vi "Preview_Build.vi"(8 "error in (no error)":errorcluster, 11 "Build in":refnum<class "AB_Targetfile.lvclass">) -> (0 "error out":errorcluster, 1 "GeneratedFiles":path[](array[path]), 3 "Build out":refnum<class "AB_Targetfile.lvclass">, 4 "GeneratedFileGUIDs":string[](array[string]), 5 "OutputDirectory":path)   [LabVIEW 2020, in "AB_Targetfile.lvclass"]
uses:
  <vilib>/AppBuilder/AB_Classes/TargetFile/AB_Targetfile.lvclass
  e:/builds/penguin/labview/branches/2020/dev/dist/vi.lib/AppBuilder/AB_Classes/Build/AB_Build.lvclass
  <vilib>/AppBuilder/AB_Classes/Build/AB_Build.lvclass
  <vilib>/AppBuilder/AB_Classes/Destination/AB_Destination.lvclass
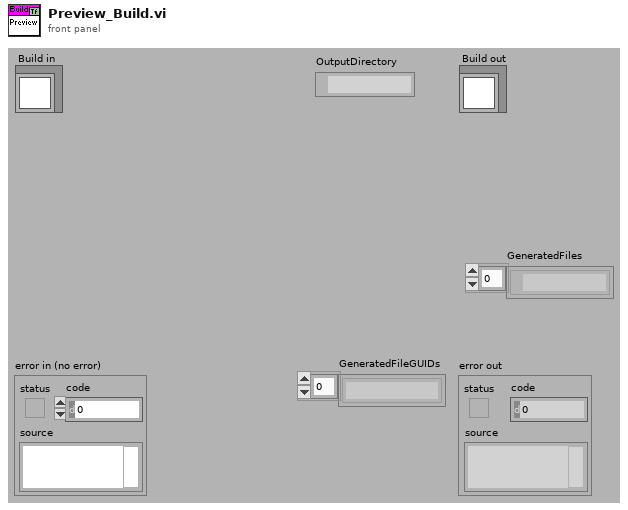
[diagram p1: front panel]
types:
  T1 = enum32{"invalid OS target", "Mac OS", "Windows 3.1", "Windows 95/NT", "Solaris 1", "Solaris 2", "HP-UX", "PowerMAX", "Linux", "Irix", "Rhapsody", "BeOS", "AIX", "OSF1", "VxWorks", "PharLap", "Carbon", "RTX", "Windows x64", "Linux x64", "Mac OS X x64"}
  T2 = typedef "AB_Build.ctl" = cluster{"buildSpecName":string, "buildSpecDescription":string, "destinations":refnum<class "AB_Destination.lvclass">[], "exclusionOption":T3, "defaultLanguage":string, "supportedLanguages":string[], "excludedDirectories":path[], "buildContext":refnum<vi>, "buildObject":T4, "preview":bool, "programatic":bool, "progressBarEvents":T5, "userLog_Path":path, "preActionID":string, "preAction_Path":path, "postActionID":string, "postAction_Path":path, "eng_checkForBrokenVIs?":bool, "eng_verboseLinkerErrors?":bool, "localDest_Path":path, "targetDest_Path":path, "removeVIObject":u16, "cache":refnum<class "PreviewCache.lvclass">, "use cache":bool, "previewCache_ID":string, "buildCache_ID":string, "eng_TempLocalDest_Path":path, "eng_collectDependencies?":bool, "versionInfo":cluster{"buildVersion":cluster{"major":u16, "minor":u16, "patch":u16, "build":u16}, "autoIncrement":bool}, "eng_enableVIChecksums":bool}
  T3 = typedef "AB_Exclusion_Option.ctl" = cluster{"typedefs":bool, "polymorphicVIs":bool, "unusedLibraryItems":bool, "modifyLibraryFile":bool, "edit-timeDependencies":bool, "inlineVIs":bool, "dependent PPLs":bool, "dependent DLLs":bool}
  T4 = typedef "ItemRef.ctl" = u64
  T5 = typedef "provcom_ProgressBar_Events.ctl" = cluster{"newJob":refnum<user-event>, "newItem":refnum<user-event>, "errorMsg":T6, "cancel":refnum<user-event>}
  T6 = typedef "mxLvBuildError.ctl" = refnum<user-event>
  T7 = typedef "AB_Destination.ctl" = cluster{"destName":string, "path":path, "libraryName":string, "preserveHierarchy":bool, "eng_inBuild":bool, "eng_libraryReference":refnum<vi>, "eng_restictAddToNewLibrary":bool}
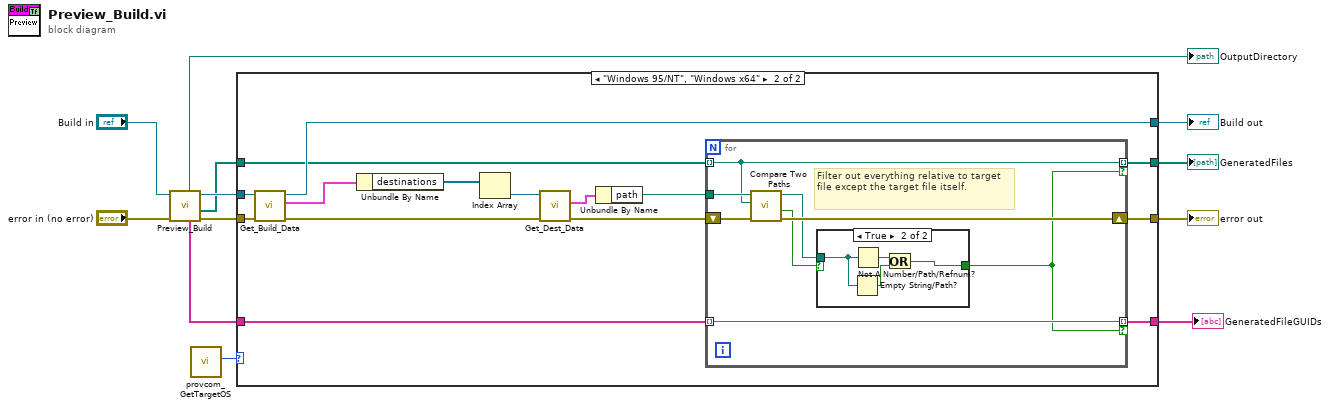
[diagram p0: block diagram]
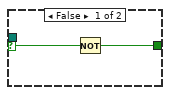
[diagram p3: hidden frame]
diagram:
  n1 = call-parent "Preview_Build.vi"("error in (no error)"="error in (no error)", "Build in"="Build in") -> ("error out"=w7:errorcluster, "GeneratedFiles"=w5:path[], "Build out"=w9:refnum<class "AB_Targetfile.lvclass">, "GeneratedFileGUIDs"=w2:string[], "OutputDirectory"=→"OutputDirectory":path)  [unwired: 5 in]
  n2 = call <resource>:"provcom_GetTargetOS.vi"() -> ("App.TargetOS"=w1:T1)  [unwired: 11 out]
  n3 = case shown="\"Windows 95/NT\", \"Windows x64\"" w1 {
    tunnel: w9 -> [w16 w31]
    tunnel: [w16 w30] -> w8
    tunnel: w7 -> [w14 w29]
    tunnel: [w14 w21] -> w6
    tunnel: w5 -> [w15 w20]
    tunnel: [w15 w19] -> w4
    tunnel: [w13 w18] -> w3
    tunnel: w2 -> [w13 w17]
    frame Default {
    }
    frame "Windows 95/NT", "Windows x64" {
      n4 = call <vilib>:"Get_Build_Data.vi"("error in (no error)"=w29, "Class in"=w31) -> ("error out"=w25:errorcluster, "data"=w28:T2, "Class out"=w30:refnum<class "AB_Targetfile.lvclass">)  [unwired: 7 in]
      n5 = Unbundle By Name(w28) -> ("destinations"=w27:refnum<class "AB_Destination.lvclass">[])
      n6 = Index Array(array=w27) -> (element=w26:refnum<class "AB_Destination.lvclass">)  [unwired: 1 in]
      n7 = call <vilib>:"Get_Dest_Data.vi"("error in (no error)"=w25, "Class in"=w26) -> ("error out"=w22:errorcluster, "destName"=w24:T7)  [unwired: 7 in, 1 out]
      n8 = Unbundle By Name(w24) -> ("path"=w23:path)
      n9 = for {
        tunnel: w23 -> [w39]
        shift-right: [w37] -> w21
        shift-left: w22 -> [w38]
        tunnel: w20 -> [w36] mode=indexing
        tunnel: [w36] -> w19 mode=indexing if=w32
        tunnel: w17 -> [w33] mode=indexing
        tunnel: [w33] -> w18 mode=indexing if=w32
        # "Filter out everything relative to target file except the target file itself."
        n10 = call <vilib>:"Compare Two Paths.vi"("error in (no error)"=w38, "Path 2"=w36, "Path 1"=w39) -> ("error out"=w37:errorcluster, "Path 2 Relative to Path 1?"=w34:bool, "Relative Path from 1 to 2"=w35:path)  [unwired: 5 in, 1 out]
        n11 = case shown="True" w34 {
          selector: w34 -> [w41 _]
          tunnel: w35 -> [_ w45]
          tunnel: [w40 w42] -> w32
          frame False {
            n12 = Not(x=w41) -> (.not. x?=w40:bool)
          }
          frame True {
            n13 = Empty String/Path?(string/path=w45) -> (empty?=w43:bool)
            n14 = Not A Number/Path/Refnum?(number/path/refnum=w45) -> (NaN/Path/Refnum?=w44:bool)
            n15 = Or(x=w44, y=w43) -> (x .or. y?=w42:bool)
          }
        }
      }
    }
  }
  "error out" <- w6
  "Build out" <- w8
  "GeneratedFiles" <- w4
  "GeneratedFileGUIDs" <- w3
